vi "Set Cells (1D Row Timestamp).vi"(6 "Column":i32, 7 "Values":timestamp[](array[timestamp]), 8 "error in (no error)":errorcluster, 9 "Row":i32, 10 "Sheet Reference":refnum<k24>) -> (0 "error out":errorcluster, 2 "Sheet Reference out":refnum<k24>)   [LabVIEW 2013]
uses:
  C:/PhaeronGit/LVNPOI/Resources/NPOI 2.1.1 dotnet2/NPOI.dll
  Resources/NPOI 2.1.1 dotnet2/NPOI.dll
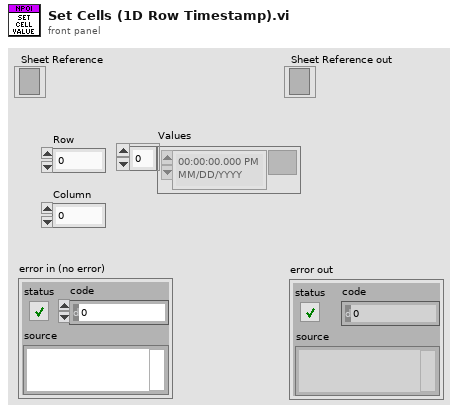
[diagram p1: front panel]
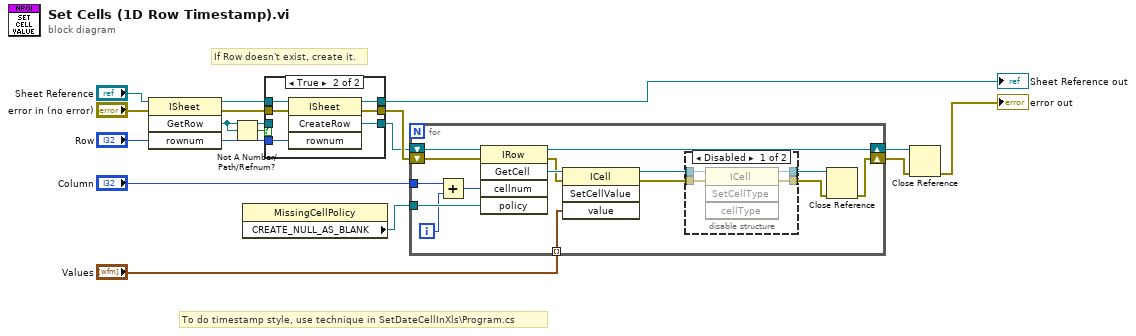
[diagram p0: block diagram]
diagram:
  # "To do timestamp style, use technique in SetDateCellInXls\\Program.cs"
  # "If Row doesn't exist, create it."
  n1 = invoke class="ISheet" method="GetRow"(reference="Sheet Reference", error in="error in (no error)", "rownum"="Row") -> (reference out=w9:refnum<k24>, error out=w10:errorcluster, "GetRow"=w12:refnum<k24>)  [unwired: 1 in, 1 out]
  n2 = Not A Number/Path/Refnum?(number/path/refnum=w12) -> (NaN/Path/Refnum?=w11:bool)
  n3 = property class="MissingCellPolicy"() -> ("CREATE_NULL_AS_BLANK"=w2:refnum<k24>)  [unwired: 2 in, 2 out]
  n4 = case shown="True" w11 {
    tunnel: w9 -> [w19 w25]
    tunnel: w10 -> [w18 w24]
    tunnel: [w18 w23] -> w4
    tunnel: [w19 w22] -> w5
    tunnel: "Row" -> [_ w21]
    tunnel: [w17 w20] -> w3
    tunnel: w12 -> [w17 _]
    frame False {
    }
    frame True {
      n5 = invoke class="ISheet" method="CreateRow"(reference=w25, error in=w24, "rownum"=w21) -> (reference out=w22:refnum<k24>, error out=w23:errorcluster, "CreateRow"=w20:refnum<k24>)  [unwired: 1 in, 1 out]
    }
  }
  "Sheet Reference out" <- w5
  n6 = for {
    tunnel: "Column" -> [w39]
    tunnel: w2 -> [w33]
    shift-right: [w40] -> w16
    shift-left: w3 -> [w34]
    shift-right: [w36] -> w14
    shift-left: w4 -> [w35]
    tunnel: "Values" -> [w32] mode=indexing
    i -> [w30]
    n7 = Add(x=w39, y=w30) -> (x+y=w31:i32)
    n8 = invoke class="IRow" method="GetCell"(reference=w34, error in=w35, "cellnum"=w31, "policy"=w33) -> (reference out=w40:refnum<k24>, error out=w37:errorcluster, "GetCell"=w38:refnum<k24>)  [unwired: 1 in, 2 out]
    n9 = invoke class="ICell" method="SetCellValue"(reference=w38, error in=w37, "value"=w32) -> (reference out=w29:refnum<k24>, error out=w28:errorcluster)  [unwired: 1 in, 2 out]
    n10 = disable-structure shown="Disabled" {
      disable-tunnel: w29 -> [w44 w46]
      disable-tunnel: w28 -> [w43 w45]
      disable-tunnel: [w42 w46] -> w27
      disable-tunnel: [w41 w45] -> w26
      frame Disabled {
        n11 = invoke class="ICell" method="SetCellType"(reference=w44, error in=w43) -> (reference out=w42:refnum<k24>, error out=w41:errorcluster)  [unwired: 2 in, 2 out]
      }
      frame Enabled {
      }
    }
    n12 = Close Reference(reference=w27, error in (no error)=w26) -> (error out=w36:errorcluster)
  }
  n13 = Close Reference(reference=w16, error in (no error)=w14) -> (error out=→"error out":errorcluster)
